vi "tsapp_transmit_can_sync_win32.vi"(5 "AAppChannel":i32(ring) items=["CHN1", "CHN2", "CHN3", "CHN4", "CHN5", "CHN6", "CHN7", "CHN8", "CHN9", "CHN10", "CHN11", "CHN12", "CHN13", "CHN14", "CHN15", "CHN16", "CHN17", "CHN18", "CHN19", "CHN20", "CHN21", "CHN22", "CHN23", "CHN24", "CHN25", "CHN26", "CHN27", "CHN28", "CHN29", "CHN30", "CHN31", "CHN32"], 7 "数据帧信息":T1 {"ADLC" max=64; "AID" max=536870911}, 11 "错误输入（无错误）":errorcluster) -> (6 "tsapp_transmit_can_sync":i32, 8 "TxOK?":bool, 15 "错误输出":errorcluster)   [LabVIEW 2016]
uses:
  Ctrl/CAN_FrameInfo.ctl
  SendMsgInfo.ctl
  TCANProperty.ctl
  TSMaster.dll
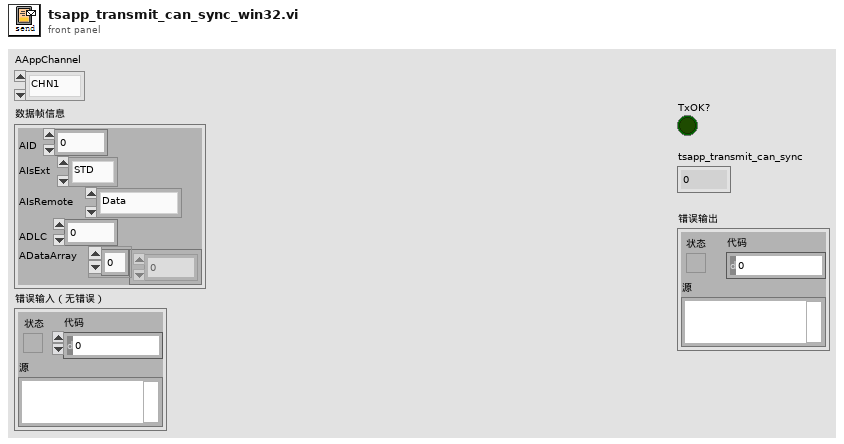
[diagram p1: front panel]
types:
  T1 = typedef "CAN_FrameInfo.ctl" = cluster{"AID":u32, "AIsExt":enum16{"STD", "EXT"}, "AIsRemote":enum16{"Data", "Remote"}, "ADLC":u8, "ADataArray":u8[]}
  T2 = typedef "TCANProperty.ctl" = cluster{"istx":bool, "remoteframe":bool, "extframe":bool, "tbd1":bool, "tbd2":bool, "tbd3":bool, "tbd4":bool, "iserrorframe":bool}
  T3 = typedef "SendMsgInfo.ctl" = cluster{"FIdxChn":u8, "FProperties":u8, "FDLC":u8, "FReserved":u8, "FIdentifier":i32, "FTimeUS":u64, "Data0":u8, "Data1":u8, "Data2":u8, "Data3":u8, "Data4":u8, "Data5":u8, "Data6":u8, "Data7":u8}
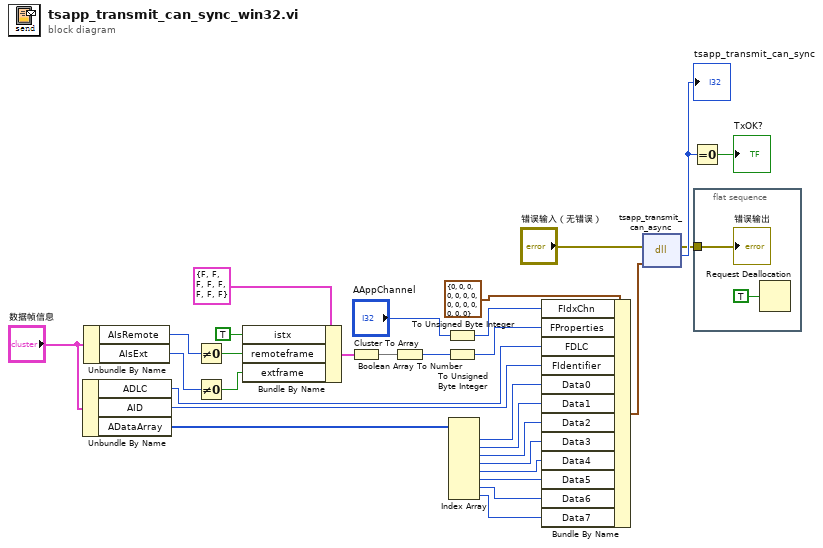
[diagram p0: block diagram]
diagram:
  n1 = Unbundle By Name("数据帧信息") -> ("ADLC"=w11:u8, "AID"=w10:u32, "ADataArray"=w9:u8[])
  n2 = Unbundle By Name("数据帧信息") -> ("AIsRemote"=w18:enum16{"Data", "Remote"}, "AIsExt"=w16:enum16{"STD", "EXT"})
  n3 = Not Equal To 0?(x=w18) -> (x != 0?=w19:bool)
  n4 = Not Equal To 0?(x=w16) -> (x != 0?=w17:bool)
  n5 = Bundle By Name(cluster=T2 {"istx"=FALSE, "remoteframe"=FALSE, "extframe"=FALSE, "tbd1"=FALSE, "tbd2"=FALSE, "tbd3"=FALSE, "tbd4"=FALSE, "iserrorframe"=FALSE} ("TCANProperty"), "istx"=TRUE, "remoteframe"=w19, "extframe"=w17) -> (w15:T2)
  n6 = Cluster To Array(cluster=w15) -> (array=w14:bool[])
  n7 = Boolean Array To Number(Boolean array=w14) -> (number=w13:u32)
  n8 = To Unsigned Byte Integer(number="AAppChannel") -> (unsigned 8bit integer=w22:u8)
  n9 = To Unsigned Byte Integer(number=w13) -> (unsigned 8bit integer=w12:u8)
  n10 = Index Array(array=w9) -> (element #1=w8:u8, element #2=w7:u8, element #3=w6:u8, element #4=w5:u8, element #5=w4:u8, element #6=w3:u8, element #7=w2:u8, element #8=w1:u8)  [unwired: 8 in]
  n11 = Bundle By Name(cluster=T3 {"FIdxChn"=0, "FProperties"=0, "FDLC"=0, "FReserved"=0, "FIdentifier"=0, "FTimeUS"=0, "Data0"=0, "Data1"=0, "Data2"=0, "Data3"=0, "Data4"=0, "Data5"=0, "Data6"=0, "Data7"=0} ("SendMsgInfo"), "FIdxChn"=w22, "FProperties"=w12, "FDLC"=w11, "FIdentifier"=w10, "Data0"=w8, "Data1"=w7, "Data2"=w6, "Data3"=w5, "Data4"=w4, "Data5"=w3, "Data6"=w2, "Data7"=w1) -> (w23:T3)
  n12 = dll-call lib="C:/Users/Eric/Desktop/LabVIEW/TSMasterAPI/Win32/CANopen_TS_2015/TSMaster.dll" fn="tsapp_transmit_can_async"(error in="错误输入（无错误）", "ACAN"=w23) -> (error out=w28:errorcluster, "tsapp_transmit_can_async"=w30:i32)  [unwired: 3 in, 1 out]
  "tsapp_transmit_can_sync" <- w30
  n13 = Equal To 0?(x=w30) -> (x = 0?=→"TxOK?":bool)
  n14 = flat-sequence {
    tunnel: w28 -> [w31]
    frame #0 {
      n15 = Request Deallocation(TRUE ("标志")) -> ()
      "错误输出" <- w31
    }
  }
